vi "KGN Set Pump Mode general.vi"(7 "PumpModeGeneral-Cluster":T3 {"dry mode" items=["wet", "dry"]; "control mode" items=["static", "pid"]}, 8 "Fehler (Eingang, kein Fehler)":errorcluster, 9 "Info Cluster":T4, 10 "VISA-Referenz (Eingang)":refnum<visa-resource-name>, 11 "device (Eingang)":u32) -> (0 "Fehler (Ausgang)":errorcluster, 1 "Info Cluster out":T4, 2 "VISA-Referenz (Ausgang)":refnum<visa-resource-name>, 3 "dup device (Ausgang)":u32, 4 "Kommandos gesendet":string)   [LabVIEW 2020, in "Linearisierung v2.lvlib" / "Gasteiler.lvlib" / "HovaCAL_Interface.lvlib" / "KGN.lvlib" / "KGN GUI Set.lvlib"]
uses:
  KGN GUI Set.lvlib
  Controls/Info Cluster.ctl
  Controls/Pump Dry Mode.ctl
  Controls/Pump Control Mode.ctl
  set/set.lvlib
  Controls/Controls.lvlib
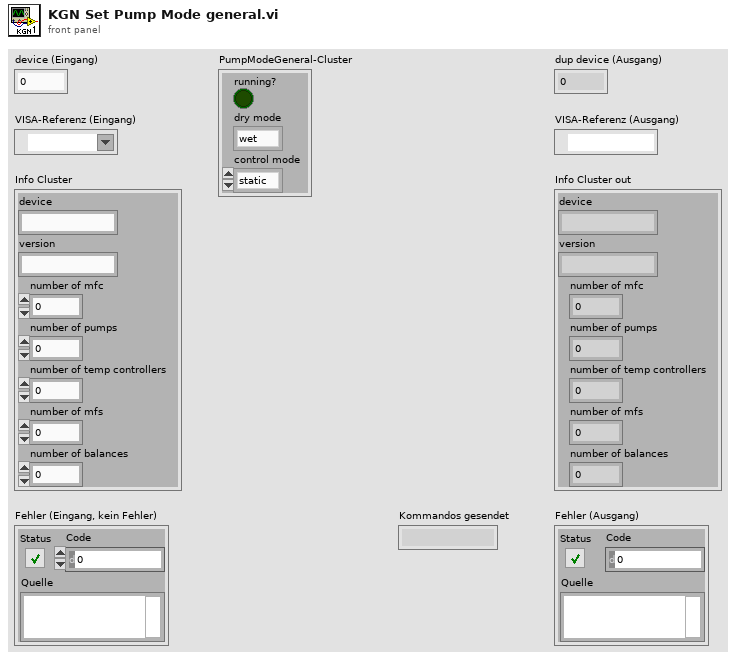
[diagram p1: front panel]
types:
  T1 = typedef "Linearisierung v2.lvlib/Gasteiler.lvlib/HovaCAL_Interface.lvlib/Controls.lvlib/Pump Dry Mode.ctl" = i32
  T2 = typedef "Linearisierung v2.lvlib/Gasteiler.lvlib/HovaCAL_Interface.lvlib/Controls.lvlib/Pump Control Mode.ctl" = u32
  T3 = cluster{"running?":bool, "dry mode":T1, "control mode":T2}
  T4 = typedef "Linearisierung v2.lvlib/Gasteiler.lvlib/HovaCAL_Interface.lvlib/Controls.lvlib/Info Cluster.ctl" = cluster{"device":string, "version":string, "number of mfc":i32, "number of pumps":i32, "number of temp controllers":i32, "number of mfs":i32, "number of balances":i32}
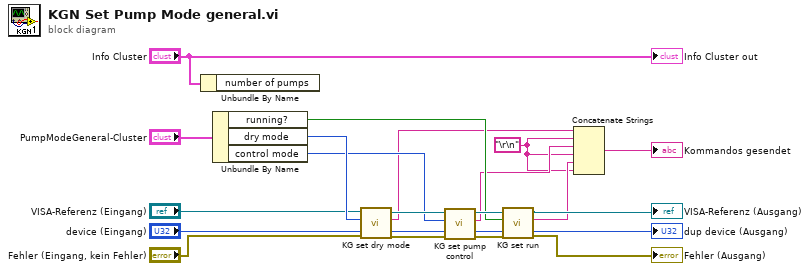
[diagram p0: block diagram]
diagram:
  w2 = "\r\n"
  n1 = Unbundle By Name("Info Cluster") -> ()  [unwired: 1 out]
  n2 = Unbundle By Name("PumpModeGeneral-Cluster") -> ("running?"=w6:bool, "dry mode"=w15:T1, "control mode"=w11:T2)
  n3 = call "KG set dry mode.vi"("Fehler (Eingang, kein Fehler)"="Fehler (Eingang, kein Fehler)", "drywet"=w15, "VISA-Ressourcenname"="VISA-Referenz (Eingang)") -> ("Fehler (Ausgang)"=w12:errorcluster, "Komando gesendet"=w5:string, "VISA-Ressourcenname (Ausgang)"=w13:refnum<visa-resource-name>)  [unwired: 6 in]
  n4 = call "KG set pump control.vi"("Fehler (Eingang, kein Fehler)"=w12, "control mode"=w11, "VISA-Ressourcenname"=w13) -> ("Fehler (Ausgang)"=w8:errorcluster, "Komando gesedet"=w4:string, "VISA-Ressourcenname (Ausgang)"=w10:refnum<visa-resource-name>)  [unwired: 6 in]
  n5 = call "KG set run.vi"("Fehler (Eingang, kein Fehler)"=w8, "run"=w6, "VISA-Ressourcenname"=w10) -> ("Fehler (Ausgang)"=→"Fehler (Ausgang)":errorcluster, "Kommando gesendet"=w3:string, "VISA-Ressourcenname (Ausgang)"=→"VISA-Referenz (Ausgang)":refnum<visa-resource-name>)  [unwired: 6 in]
  n6 = Concatenate Strings(w5, w2, w4, w2, w3, w2) -> (→"Kommandos gesendet":string)
  "dup device (Ausgang)" <- "device (Eingang)"
  "Info Cluster out" <- "Info Cluster"
